vi "Send Asynchronous Message.vi"(8 "error in (no error)":errorcluster, 10 "Async Message":refnum<class "Async Message.lvclass">, 11 "1553 Component in":refnum<class "1553 Component.lvclass">) -> (0 "error out":errorcluster, 3 "1553 Component out":refnum<class "1553 Component.lvclass">)   [LabVIEW 2020, in "BCI-1553 API.lvlib" / "1553 Component.lvclass"]
doc: "If this component is configured as a Bus Controller, this method will send an asynchronous message out on the bus as soon as possible and add the asynchronous message parameters to this component."
uses:
  1553 Component.lvclass
  Frames & Messages/Async Message/Async Message.lvclass
  1553 Component.lvclass/1553 Component.ctl
  Bus Controller/Bus Controller.lvclass
  C:/Users/MattJ/Desktop/git/bci-1553-labview-api/src/1553 SubComponent/1553 SubComponent.lvclass
  1553 SubComponent/1553 SubComponent.lvclass
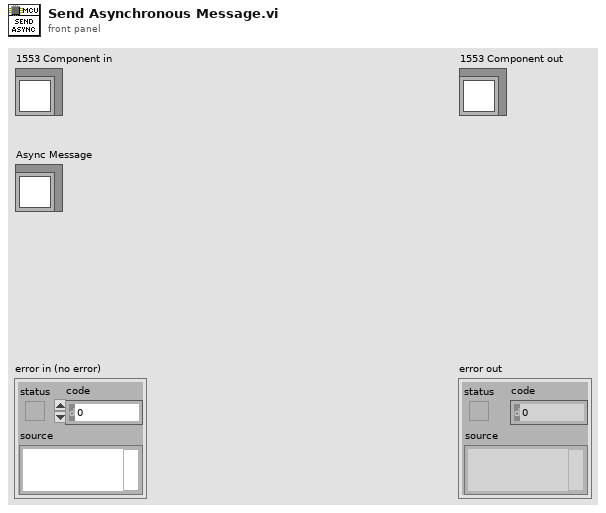
[diagram p1: front panel]
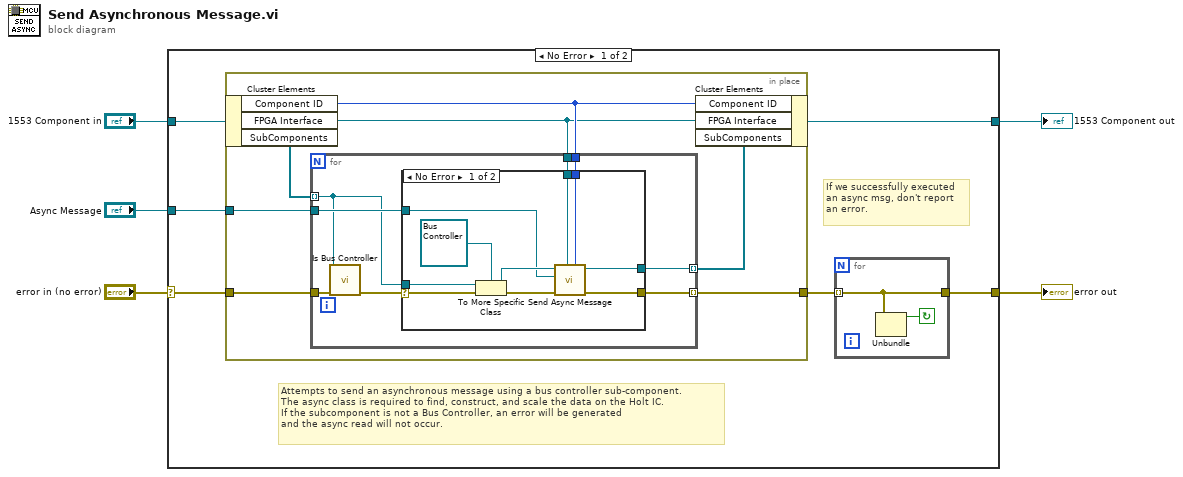
[diagram p0: block diagram]
diagram:
  n1 = case shown="No Error" "error in (no error)" {
    selector: "error in (no error)" -> [w9 w42]
    tunnel: [w7 w42] -> w1
    tunnel: [w10 w41] -> w2
    tunnel: "1553 Component in" -> [w11 w41]
    tunnel: "Async Message" -> [w8 _]
    frame No Error {
      # "If we successfully executed\nan async msg, don't report\nan error."
      # "Attempts to send an asynchronous message using a bus controller sub-component.\nThe async class is required to find, construct, and scale the data on the Holt IC.\nIf the subcomponent is not a Bus Controller, an error will be generated\nand the async read will not occur."
      n2 = in-place {
        in-place-border: w9 -> [w16]
        in-place-border: [w14] -> w6
        in-place-border: w8 -> [w15]
        n3 = in-place-cluster #1(w11) -> ("Component ID"=w20:u8, "FPGA Interface"=w17:refnum<class "FPGA Interface.lvclass">, "SubComponents"=w19:refnum<class "1553 SubComponent.lvclass">[])
        n4 = for {
          tunnel: w19 -> [w21] mode=indexing
          tunnel: [w26] -> w18 mode=indexing
          tunnel: w20 -> [w28]
          tunnel: w17 -> [w27]
          tunnel: w16 -> [w24]
          tunnel: [w25] -> w14 mode=indexing
          tunnel: w15 -> [w22]
          n5 = call "Is Bus Controller.vi"("error in (no error)"=w24, "1553 SubComponent"=w21) -> ("error out"=w23:errorcluster)  [unwired: 9 in]
          n6 = case shown="No Error" w23 {
            selector: w23 -> [w37 w39]
            tunnel: w28 -> [w34 _]
            tunnel: w27 -> [w35 _]
            tunnel: [w31 w40] -> w26
            tunnel: [w30 w39] -> w25
            tunnel: w21 -> [w38 w40]
            tunnel: w22 -> [w32 _]
            frame No Error {
              n7 = To More Specific Class(target class=refnum<class "Bus Controller.lvclass"> refnum ("SLSC 1553 API.lvlib:Bus Controller.lvclass"), reference=w38, error in=w37) -> (specific class reference=w33:refnum<class "Bus Controller.lvclass">, error out=w29:errorcluster)
              n8 = call-dynamic "Send Async Message.vi"("Component ID"=w34, "FPGA Interface"=w35, "error in (no error)"=w29, "Async Message"=w32, "Bus Controller in"=w33) -> ("error out"=w30:errorcluster, "Bus Controller out"=w31:refnum<class "Bus Controller.lvclass">)  [unwired: 5 in]
            }
            frame Error {
            }
          }
        }
        n9 = in-place-cluster #1("Component ID"=w20, "FPGA Interface"=w17, "SubComponents"=w18) -> (w10:refnum<class "1553 Component.lvclass">)
      }
      n10 = for {
        tunnel: [w13] -> w7
        tunnel: w6 -> [w13] mode=indexing
        stop <- w12 continue-if-true
        n11 = Unbundle(w13) -> ("status"=w12:bool)  [unwired: 2 out]
      }
    }
    frame Error {
    }
  }
  "error out" <- w1
  "1553 Component out" <- w2
